vi "IsAntsRectValid.vi"(11 "AntsRect":T1) -> (3 "Valid?":bool, 5 "Max. Rect size?":bool)   [LabVIEW 2020]
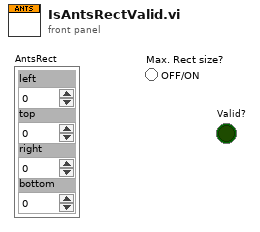
[diagram p1: front panel]
types:
  T1 = cluster{"left":i16, "top":i16, "right":i16, "bottom":i16}
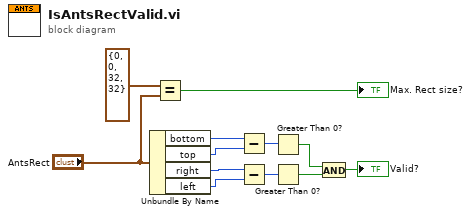
[diagram p0: block diagram]
diagram:
  n1 = Unbundle By Name("AntsRect") -> ("bottom"=w12:i16, "top"=w11:i16, "right"=w10:i16, "left"=w9:i16)
  n2 = Equal?(x=T1 {"left"=0, "top"=0, "right"=32, "bottom"=32}, y="AntsRect") -> (x = y?=→"Max. Rect size?":bool)
  n3 = Subtract(x=w12, y=w11) -> (x-y=w8:i16)
  n4 = Subtract(x=w10, y=w9) -> (x-y=w7:i16)
  n5 = Greater Than 0?(x=w8) -> (x > 0?=w5:bool)
  n6 = Greater Than 0?(x=w7) -> (x > 0?=w6:bool)
  n7 = And(x=w5, y=w6) -> (x .and. y?=→"Valid?":bool)
